vi "Send Event Based Assert.vi"(8 "error in (no error)":errorcluster, 11 "Assert Message in":T1) -> (0 "error out":errorcluster)   [LabVIEW 2017, in "Assert API Components.lvlib" / "Log Assert Core.lvlib"]
doc: "Sends an assert message using the user event based method - should be more reliable and higher performance than the network comms method, but is restricted to LV dev environment on Windows only."
uses:
  Log Assert Core.lvlib
  Message Data.ctl
  Failure Actions.ctl
  Assert Event Actions.ctl
  Assert API Components.lvlib
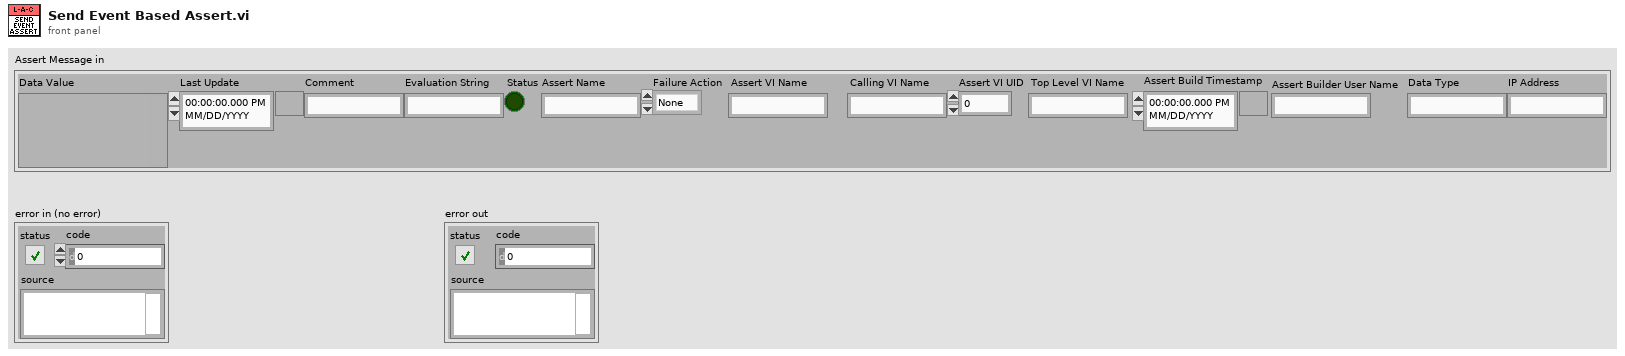
[diagram p1: front panel]
types:
  T1 = typedef "Assert API Components.lvlib/Message Data.ctl" = cluster{"Data Value":variant, "Last Update":timestamp, "Comment":string, "Evaluation String":string, "Status":bool, "Assert Name":string, "Failure Action":T2, "Assert VI Name":string, "Calling VI Name":string, "Assert VI UID":i32, "Top Level VI Name":string, "Assert Build Timestamp":timestamp, "Assert Builder User Name":string, "Data Type":string, "IP Address":string}
  T2 = typedef "Assert API Components.lvlib/Failure Actions.ctl" = enum16{"None", "Log To File", "Pause Execution", "Abort Execution"}
  T3 = typedef "Assert API Components.lvlib/Assert Event Actions.ctl" = enum16{"Init", "Read", "Destroy"}
  T4 = typedef "Assert API Components.lvlib/Log Assert Core.lvlib/Failure Action Change Event Reference.ctl" = cluster{"Failure Action Change Event":refnum<user-event>, "Event Registration Refnum":refnum<event-registration>}
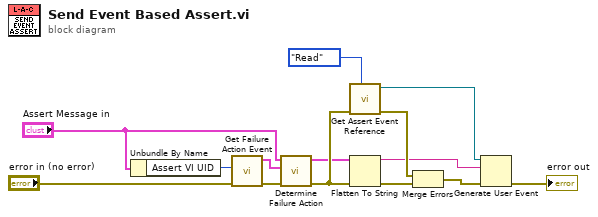
[diagram p0: block diagram]
diagram:
  n1 = Unbundle By Name("Assert Message in") -> ("Assert VI UID"=w12:i32)
  n2 = call "Get Failure Action Event.vi"("error in (no error)"="error in (no error)", "Assert VI UID"=w12) -> ("error out"=w13:errorcluster, "Failure Action Event References"=w14:T4)  [unwired: 8 in]
  n3 = call "Determine Failure Action.vi"("error in (no error)"=w13, "Failure Action Change Event References"=w14, "Assert Message in"="Assert Message in") -> ("error out"=w5:errorcluster, "Assert Message out"=w1:T1)  [unwired: 7 in]
  n4 = call "Get Assert Event Reference.vi"("Action"=Assert_Event_Actions."Read", "error in (no error)"=w5) -> ("error out"=w3:errorcluster, "Assert Message Event"=w9:refnum<user-event>)  [unwired: 8 in]
  n5 = Flatten To String(anything=w1, error in (no error)=w5) -> (data string=w2:string, error out=w7:errorcluster)  [unwired: 2 in, 1 out]
  n6 = Merge Errors(w3, w7) -> (w4:errorcluster)
  n7 = Generate User Event(user event=w9, event data cluster=w2, error in=w4) -> (error out=→"error out":errorcluster)  [unwired: 1 in, 1 out]
